vi "Parse Signal List.vi"(8 "error in":errorcluster, 11 "Electronic Load in":refnum<class "Electronic Load.lvclass">) -> (0 "error out":errorcluster, 3 "Electronic Load out":refnum<class "Electronic Load.lvclass">)   [LabVIEW 2019, in "Electronic Load.lvlib" / "Electronic Load.lvclass"]
uses:
  Library/Electronic Load.lvclass
  C:/Users/Public/Documents/Development/builds/Tools/Config.lvlibp/Config.lvclass
  Library/Electronic Load.lvclass/Electronic Load.ctl
  Accessors/Read Available Channels.vi
  builds/Tools/Config.lvlibp/Accessors/Read Device Signals.vi
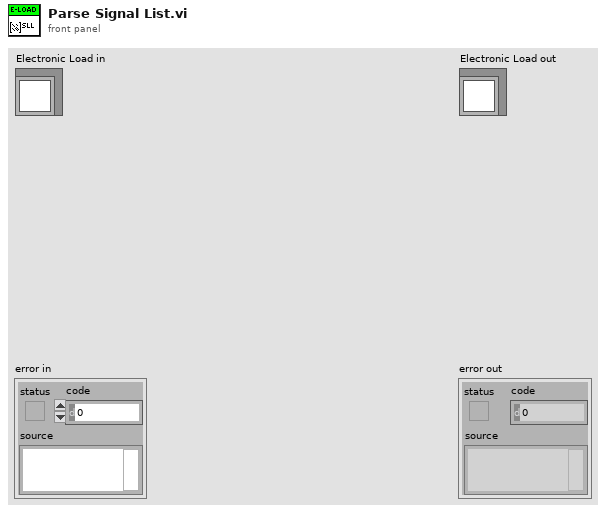
[diagram p1: front panel]
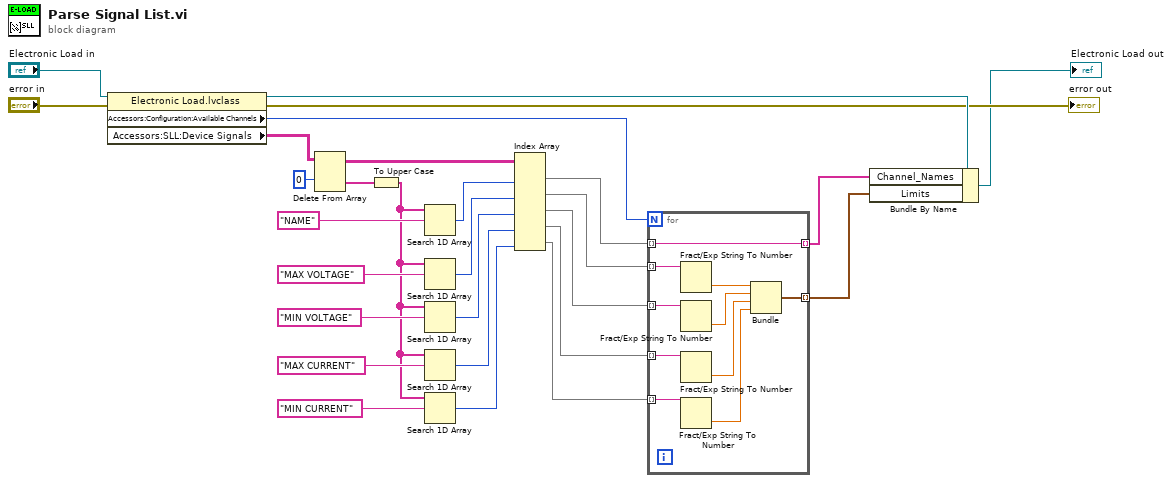
[diagram p0: block diagram]
diagram:
  n1 = property class="Electronic Load.lvclass"(reference="Electronic Load in", error in="error in") -> (reference out=w26:refnum<class "Electronic Load.lvclass">, error out=→"error out":errorcluster, "Accessors:Configuration:Available Channels"=w1:i32, "Accessors:SLL:Device Signals"=w24:string[][])
  n2 = Delete From Array(array=w24, index (row)=0) -> (deleted portion=w21:string[], array with subset deleted=w20:string[][])  [unwired: 2 in]
  n3 = To Upper Case(1:w21) -> (0:w13:string[])
  n4 = Search 1D Array(1D array=w13, element="NAME") -> (index of element=w19:i32)  [unwired: 1 in]
  n5 = Search 1D Array(1D array=w13, element="MAX VOLTAGE") -> (index of element=w12:i32)  [unwired: 1 in]
  n6 = Search 1D Array(1D array=w13, element="MIN VOLTAGE") -> (index of element=w11:i32)  [unwired: 1 in]
  n7 = Search 1D Array(1D array=w13, element="MAX CURRENT") -> (index of element=w10:i32)  [unwired: 1 in]
  n8 = Search 1D Array(1D array=w13, element="MIN CURRENT") -> (index of element=w9:i32)  [unwired: 1 in]
  n9 = Index Array(array=w20, index (col) #1=w19, index (col) #2=w12, index (col) #3=w11, index (col) #4=w10, index (col) #5=w9) -> (element #1=w3:string[], element #2=w8:string[], element #3=w7:string[], element #4=w6:string[], element #5=w5:string[])  [unwired: 5 in]
  n10 = for {
    N: w1 -> [_]
    tunnel: w8 -> [w38] mode=indexing
    tunnel: w7 -> [w37] mode=indexing
    tunnel: w6 -> [w35] mode=indexing
    tunnel: w5 -> [w36] mode=indexing
    tunnel: [w30] -> w4 mode=indexing
    tunnel: w3 -> [w29] mode=indexing
    tunnel: [w29] -> w2 mode=indexing
    n11 = Fract/Exp String To Number(string=w38) -> (number=w34:dbl)  [unwired: 3 in, 1 out]
    n12 = Fract/Exp String To Number(string=w37) -> (number=w33:dbl)  [unwired: 3 in, 1 out]
    n13 = Fract/Exp String To Number(string=w35) -> (number=w32:dbl)  [unwired: 3 in, 1 out]
    n14 = Fract/Exp String To Number(string=w36) -> (number=w31:dbl)  [unwired: 3 in, 1 out]
    n15 = Bundle(w34, w33, w32, w31) -> (w30:cluster{dbl, dbl, dbl, dbl})  [unwired: 1 in]
  }
  n16 = Bundle By Name(cluster=w26, "Channel_Names"=w2, "Limits"=w4) -> (→"Electronic Load out":refnum<class "Electronic Load.lvclass">)
